vi "Without DRAM Packing Test Compile.vi"() -> ()   [LabVIEW 2013]
doc: "This is the FPGA VI for the 10-Tap 8-Bit Camera with DRAM example. This example demonstrates how to acquire images from a 10-tap, 8-bit, extended configuration, Camera Link camera and transfer the images to the host. This example supports area scan and line scan cameras for both continuous and finite acquisitions.\n\nThis example also demonstrates the use of DRAM as a frame buffer for very high speed acquisitions. Data packing and flow-control are also employed to maximize use of the available DRAM and FIFOs in terms of both memory space and performance.\n\nAdditionally, the example demonstrates the serial server, which allows third-party camera configuration utilities to communicate with the camera using the Camera Link serial interface while this VI is running."
uses:
  <vilib>/rvi/DataTransferAndStorage/Container/XNode/niFpgaContainer.xnode
  <vilib>/Platform/TimedLoop/XDataNode/XDataNode.xnode
  <vilib>/Platform/TimedLoop/XDataNode/timing_clust.ctl
  <vilib>/Platform/TimedLoop/XDataNode/XDNodeRunTimeDep.lvlib
  <vilib>/Platform/TimedLoop/XDataNode/wakeup.ctl
  <vilib>/Platform/TimedLoop/XDataNode/nitl_modes.ctl
  <vilib>/eio/EIONode/EIONode.xnode
  <vilib>/rvi/eio/common/nirviEmuTemplateMethod_errors.vi
  <vilib>/rvi/FIFO/Fifo_Resource/nirvififoEmulationGetNumberOfElementsToRead.vi
  <vilib>/rvi/interface/RandomDataEmulation/nirviRandomDataFpgaReadWriteTemplate.vi
  <vilib>/rvi/FIFO/Fifo_Resource/nirvififoEmulationRead.vi
  <vilib>/rvi/FIFO/Fifo_Resource/nirvififoEmulationWrite.vi
  Common/CL Data to Pixels/10 Tap 8-Bit.vi
  FPGA/10-Tap Data/10-Tap Conversion Enum.ctl
  FPGA/Globals/Accumulated Sector Intensity.vi
  FPGA/Globals/Pixel Location Global.vi
  FPGA/Globals/Wing Square Wave Frequency Global.vi
  FPGA/Globals/Sector Parameter Global.vi
  Common/CL Signal Mapping.ctl
  Common/CL Configuration.ctl
  FPGA/Sector/Accumulate/Sector Parameter Cluster.ctl
panel:
  in  "[Average BG Intensity]":u8[](array[numeric])=[0, 0, 0, 0, 0, 0, 0, 0, 0, 0, 0, 0, 0, 0, 0, 0, 0, 0, 0, 0, 0, 0, 0, 0, 0, 0, 0, 0, 0, 0, 0, 0]
  in  "Sector Threshold":u8
  in  "# of Frames to Average":u8
  in  "Sector Parameters Right":T1={"Start Angle"=0.13543701171875, "End Angle"=0.30462646484375, "Inner Radius"=309, "Outter Radius"=405, "Hinge X"=1106, "Hinge Y"=803, "NumWingSectors"=8}
  in  "Sector Parameters Left":T1={"Start Angle"=0.6541748046875, "End Angle"=0.856201171875, "Inner Radius"=309, "Outter Radius"=405, "Hinge X"=947, "Hinge Y"=829, "NumWingSectors"=8}
  in  "Sim":bool=TRUE
  in  "CL Config.Configuration":T2=enum."Full"
  in  "CL Config.Signal Mapping":T3=enum."Basler 10-tap"
  in  "CL Config.Line Scan":bool
  in  "CL Config.DVAL Active High":bool=TRUE
  in  "CL Config.LVAL Active High":bool=TRUE
  in  "CL Config.FVAL Active High":bool=TRUE
  in  "CL Config.Spare Active High":bool=TRUE
  in  "Acq Control.Line Scan Height":u32
  in  "Acq Control.Frames To Acq":u32
  in  "Acq Control.Acquire":bool
  in  "Acq Control.Cancel Acq":bool
  in  "Acq Control.Ignore DVAL":bool
  in  "Acq Control.Initialize":bool
  out "Acq Status.Acq In Progress":bool
  out "Acq Status.Clocks Per Line":u32
  out "Acq Status.Frames Acq'd":u32
  out "Acq Status.Lines Per Frame":u32
  out "Acq Status.DMA Write Timeout":bool
  out "Acq Status.Initialized":bool
  in  "UART.Baud Rate":u8
  in  "UART.Transmit":bool
  in  "UART.Tx Data":u8[](array[numeric])=[0, 0, 0, 0, 0, 0, 0, 0, 0, 0] format="%02x"
  in  "UART.Set Baud Rate":bool
  in  "UART.Byte Mode":bool=TRUE
  out "UART.Rx Ready":bool
  out "UART.Break Indicator":bool
  out "UART.Framing Error":bool
  out "UART.Overrun Error":bool
  out "UART.Tx Ready":bool
  out "UART.Rx Data":u8 format="%02x"
  in  "UART.Receive":bool
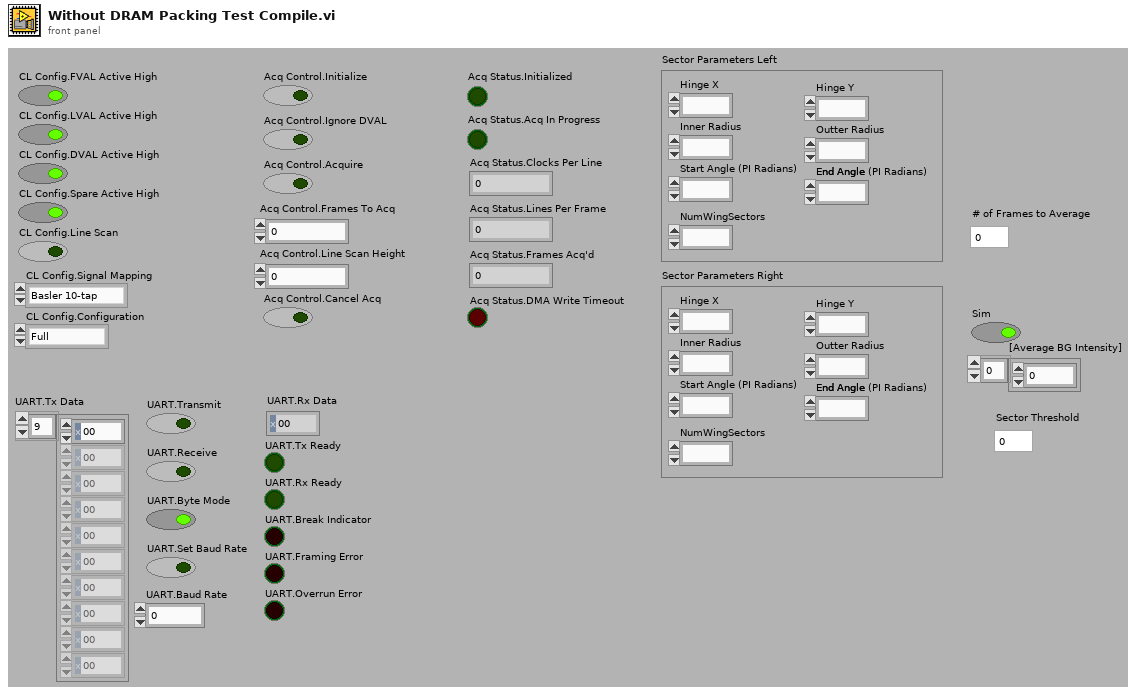
[diagram p1: front panel]
types:
  T1 = typedef "Sector Parameter Cluster.ctl" = cluster{"Start Angle":fxp<+/-,17,2>, "End Angle":fxp<+,17,3>, "Inner Radius":u16, "Outter Radius":u16, "Hinge X":u16, "Hinge Y":u16, "NumWingSectors":u8}
  T2 = typedef "CL Configuration.ctl" = enum8{"Base", "Medium", "Full"}
  T3 = typedef "CL Signal Mapping.ctl" = enum8{"Standard", "Basler 10-tap", "Vosskühler 10-tap"}
  T4 = typedef "XDNodeRunTimeDep.lvlib/timing_clust.ctl" = cluster{"Expected End [f-1]":u64, "Actual End [f-1]":u64, "Finished Late? [f-1]":bool, "Expected End [i-1]":u64, "Actual End [i-1]":u64, "Finished Late? [i-1]":bool, "Expected Start [i]":u64, "Actual Start [i]":u64, "Expected Start [f]":u64, "Actual Start [f]":u64, "Source Name":string, "Structure Name":string, "Period":i64, "Deadline":i64, "Offset":i64, "Start":i64, "Priority":i32, "Timeout":i32, "Mode":T5, "Wakeup Reason":T6, "Error":errorcluster, "Source Type":string, "Secondary Source Type":string, "Global End Time":u64, "Global Start Time":u64, "Frame Duration":u64, "Iteration Duration":u64, "Assigned CPU":i32, "I/O Scan Engine Mode":u32}
  T5 = typedef "XDNodeRunTimeDep.lvlib/nitl_modes.ctl" = enum32{"No Change", "Process missed periods, maintain original phase", "Discard missed periods, maintain original phase", "Process missed periods, ignore original phase", "Discard missed periods, ignore original phase"}
  T6 = typedef "XDNodeRunTimeDep.lvlib/wakeup.ctl" = enum32{"Normal", "Aborted", "Asynchronous wakeup", "Timing source error", "Timed loop error", "Timeout"}
  T7 = typedef "10-Tap Conversion Enum.ctl" = enum16{"10-Tap to 16 and 64", "16 and 64 to 10-Tap"}
  T8 = cluster{"Enables Valid":bool, "Frame Valid":bool, "Line Valid":bool, "Data Valid":bool}
  T9 = typedef "10-Tap 8-bit Cluster.ctl" = cluster{"Pixel 0":u8, "Pixel 1":u8, "Pixel 2":u8, "Pixel 3":u8, "Pixel 4":u8, "Pixel 5":u8, "Pixel 6":u8, "Pixel 7":u8, "Pixel 8":u8, "Pixel 9":u8}
  T10 = cluster{"Tx Data":u8[], "Transmit":bool, "Receive":bool, "Byte Mode":bool, "Set Baud Rate":bool, "Baud Rate":u8}
  T11 = cluster{"Rx Data":u8, "Turn Off Transmit":bool, "Turn Off Receive":bool, "Turn Off Set Baud Rate":bool, "Tx Ready":bool, "Rx Ready":bool, "Break Indicator":bool, "Framing Error":bool, "Overrun Error":bool}
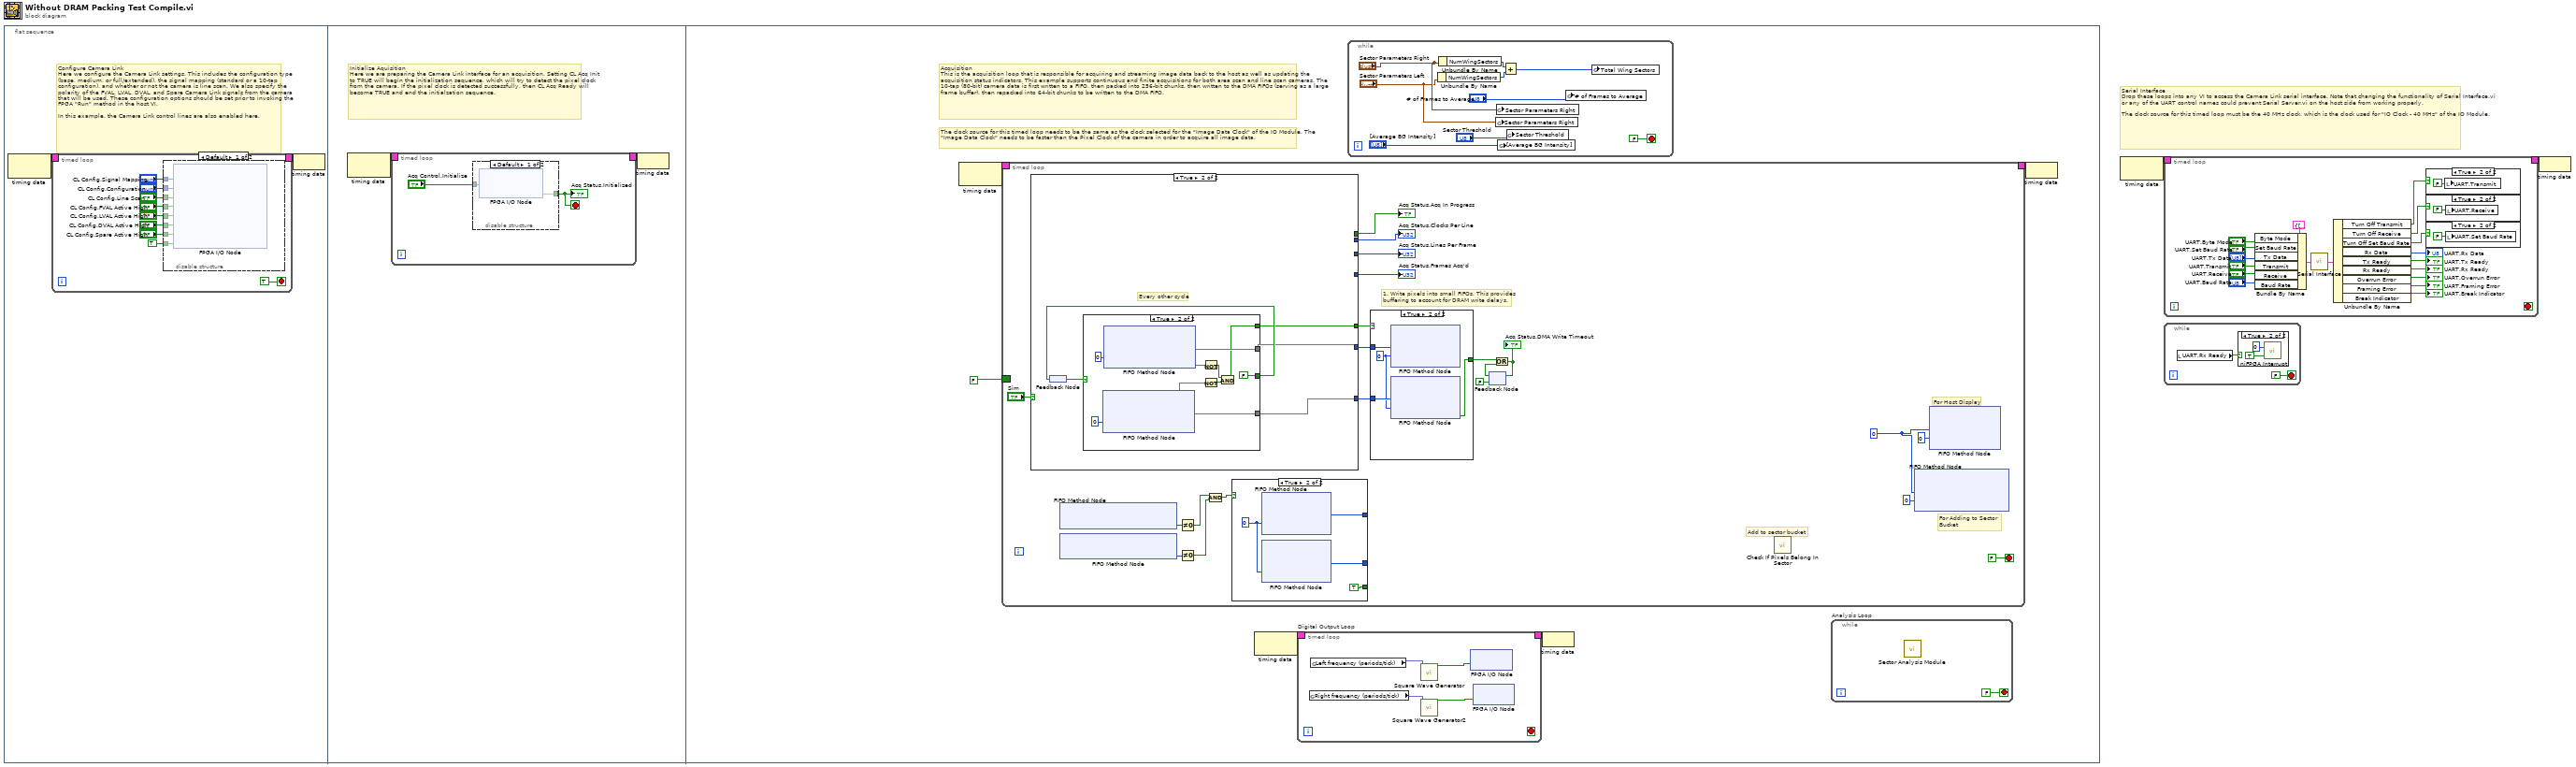
[diagram p0: block diagram]
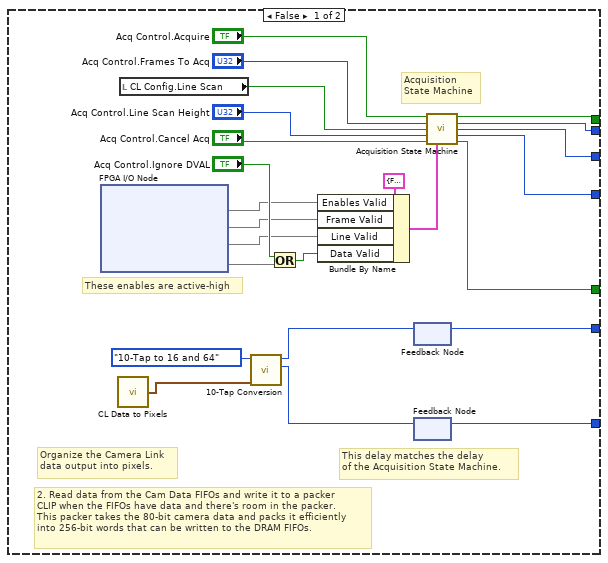
[diagram p8: hidden frame]
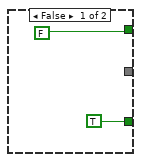
[diagram p9: hidden frame]
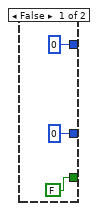
[diagram p10: hidden frame]
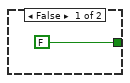
[diagram p11: hidden frame]
diagram:
  # "Serial Interface\nDrop these loops into any VI to access the Camera Link serial interface. Note that changing the functionality of Serial Interface.vi or any of the UART control names could prevent Serial Server.vi on the host side from working properly.\n\nThe clock source for this timed loop must be the 40 MHz clock, which is the clock used for \"IO Clock - 40 MHz\" of the IO Module."
  n1 = flat-sequence {
    frame #0 {
      # "Configure Camera Link\nHere we configure the Camera Link settings. This includes the configuration type (base, medium, or full/extended), the signal mapping (standard or a 10-tap configuration), and whether or not the camera is line scan. We also specify the polarity of the FVAL, LVAL, DVAL, and Spare Camera Link signals from the camera that will be used. These configuration options should be set prior to invoking the FPGA \"Run\" method in the host VI.\n\nIn this example, the Camera Link control lines are also enabled here."
      n2 = node-c288() -> (w4:T4)  [unwired: 1 in]
      n3 = timed-loop {
        timing: w4 -> [_]
        timing-out: [_] -> w3
        stop <- TRUE stop-if-true
        n4 = disable-structure shown="Default" {
          disable-tunnel: "CL Config.FVAL Active High" -> [w21 _]
          disable-tunnel: "CL Config.LVAL Active High" -> [w20 _]
          disable-tunnel: "CL Config.DVAL Active High" -> [w19 _]
          disable-tunnel: "CL Config.Spare Active High" -> [w18 _]
          disable-tunnel: "CL Config.Signal Mapping" -> [w17 _]
          disable-tunnel: "CL Config.Configuration" -> [w16 _]
          disable-tunnel: "CL Config.Line Scan" -> [w15 _]
          disable-tunnel: TRUE ("IO Module\\CL Control Enable") -> [w14 _]
          frame condition #0 {
            n5 = xnode "FPGA I/O Node"("CL Set Signal Mapping"=w17, "CL Set Configuration"=w16, "CL Set Line Scan"=w15, "CL Set FVAL Active High"=w21, "CL Set LVAL Active High"=w20, "CL Set DVAL Active High"=w19, "CL Set Spare Active High"=w18, "CL Control Enable"=w14) -> ()  [unwired: 8 in, 8 out]
          }
          frame condition #1 (active) {
          }
        }
      }
      n6 = node-c288(w3) -> ()
    }
    frame #1 {
      # "Initialize Aquisition\nHere we are preparing the Camera Link interface for an acquisition. Setting CL Acq Init to TRUE will begin the initialization sequence, which will try to detect the pixel clock from the camera. If the pixel clock is detected successfully, then CL Acq Ready will become TRUE and end the initialzation sequence."
      n7 = node-c288() -> (w27:T4)  [unwired: 1 out]
      n8 = timed-loop {
        timing: w27 -> [_]
        timing-out: [_] -> w26
        stop <- w28 stop-if-true
        n9 = disable-structure shown="Default" {
          disable-tunnel: "Acq Control.Initialize" -> [w31 w32]
          disable-tunnel: [w30 w32] -> w28
          frame condition #0 {
            n10 = xnode "FPGA I/O Node"("CL Acq Init"=w31) -> ("CL Acq Ready"=w30)  [unwired: 2 in, 2 out]
          }
          frame condition #1 (active) {
          }
        }
        "Acq Status.Initialized" <- w28
      }
      n11 = node-c288(w26) -> ()
    }
    frame #2 {
      # "The clock source for this timed loop needs to be the same as the clock selected for the \"Image Data Clock\" of the IO Module. The \"Image Data Clock\" needs to be faster than the Pixel Clock of the camera in order to acquire all image data."
      # "Acquisition\nThis is the acquisition loop that is responsible for acquiring and streaming image data back to the host as well as updating the acquisition status indicators. This example supports continuous and finite acquisitions for both area scan and line scan cameras. The 10-tap (80-bit) camera data is first written to a FIFO, then packed into 256-bit chunks, then written to the DMA FIFOs (serving as a large frame buffer), then repacked into 64-bit chunks to be written to the DMA FIFO."
      n12 = node-c288() -> (w41:T4)  [unwired: 1 in]
      n13 = timed-loop {
        timing: w41 -> [_]
        timing-out: [_] -> w40
        border: FALSE -> [_]
        stop <- FALSE stop-if-true
        w60 = u64 0 ("Element")
        # "For Adding to Sector \nBucket"
        # "For Host Display"
        # "Add to sector bucket"
        # "1. Write pixels into small FIFOs. This provides\nbuffering to account for DRAM write delays."
        n14 = case shown="True" "Sim" {
          tunnel: [w104 w105] -> w80
          tunnel: [w103 w106] -> w75
          tunnel: [w85 w108] -> w67
          tunnel: [w89 _] -> w66
          tunnel: [w88 _] -> w65
          tunnel: [w87 _] -> w64
          tunnel: [w86 _] -> w63
          frame False {
            # "These enables are active-high"
            # "Acquisition\nState Machine"
            # "2. Read data from the Cam Data FIFOs and write it to a packer\nCLIP when the FIFOs have data and there's room in the packer.\nThis packer takes the 80-bit camera data and packs it efficiently\ninto 256-bit words that can be written to the DRAM FIFOs."
            # "Organize the Camera Link\ndata output into pixels."
            # "This delay matches the delay\nof the Acquisition State Machine."
            n15 = xnode "FPGA I/O Node"() -> ("CL Output Valid"=w93, "CL Frame Valid"=w94, "CL Line Valid"=w95, "CL Data Valid"=w98)  [unwired: 4 in, 4 out]
            n16 = call-poly "CL Data to Pixels.vi"() -> ("Pixels"=w81:T9)  [unwired: 1 in]
            n17 = local read "CL Config.Line Scan"() -> (w101:bool)
            n18 = call "10-Tap Conversion.vi"("10 Tap In"=w81, "Operation"=10-Tap_Conversion_Enum."10-Tap to 16 and 64") -> ("64 Bit Out"=w82:u64, "16 Bit Out"=w83:u16)  [unwired: 7 in, 1 out]
            n19 = Or(x="Acq Control.Ignore DVAL", y=w98) -> (x .or. y?=w99:bool)
            n20 = Bundle By Name(cluster=T8 {"Enables Valid"=FALSE, "Frame Valid"=FALSE, "Line Valid"=FALSE, "Data Valid"=FALSE} ("Enables"), "Enables Valid"=w93, "Frame Valid"=w94, "Line Valid"=w95, "Data Valid"=w99) -> (w96:T8)
            n21 = feedback #1() -> (w103:u16)  [unwired: 1 in]
            n22 = feedback-in #1(w83) -> ()
            n23 = feedback #2() -> (w104:u64)  [unwired: 1 in]
            n24 = feedback-in #2(w82) -> ()
            n25 = call "Acquisition State Machine.vi"("Acquire"="Acq Control.Acquire", "Frames to Acquire"="Acq Control.Frames To Acq", "Line Scan"=w101, "Line Scan Height"="Acq Control.Line Scan Height", "Cancel Acq"="Acq Control.Cancel Acq", "Enables"=w96) -> ("Acq In Progress"=w89:bool, "Num Clocks Per Line"=w88:u32, "Num Lines Per Frame"=w87:u32, "Num Frames Acq'd"=w86:u32, "Capture Cycle"=w85:bool)  [unwired: 4 in, 1 out]
          }
          frame True {
            # "Every other cycle"
            n26 = feedback #3() -> (w107:bool)
            n27 = case shown="True" w107 {
              tunnel: [_ w121] -> w106
              tunnel: [_ w120] -> w105
              tunnel: [FALSE w113] -> w108
              tunnel: [TRUE FALSE] -> w109
              frame False {
              }
              frame True {
                n28 = xnode ("FIFO Method Node")("Timeout"=0) -> ("Element"=w120, "Timed Out?"=w116)  [unwired: 1 in, 1 out]
                n29 = xnode ("FIFO Method Node")("Timeout"=0) -> ("Element"=w121, "Timed Out?"=w117)  [unwired: 1 in, 1 out]
                n30 = Not(x=w117) -> (.not. x?=w115:bool)
                n31 = Not(x=w116) -> (.not. x?=w114:bool)
                n32 = And(x=w115, y=w114) -> (x .and. y?=w113:bool)
              }
            }
            n33 = feedback-in #3(w109) -> ()
          }
        }
        "Acq Status.Frames Acq'd" <- w63
        "Acq Status.Lines Per Frame" <- w64
        "Acq Status.Clocks Per Line" <- w65
        "Acq Status.Acq In Progress" <- w66
        n34 = xnode ("FIFO Method Node")() -> ("Number of Elements to Read"=w74:u32)  [unwired: 1 in, 1 out]
        n35 = xnode ("FIFO Method Node")() -> ("Number of Elements to Read"=w73:u32)  [unwired: 1 in, 1 out]
        n36 = Not Equal To 0?(x=w74) -> (x != 0?=w71:bool)
        n37 = Not Equal To 0?(x=w73) -> (x != 0?=w70:bool)
        n38 = Compound Arithmetic op=AND(w71, w70) -> (w72:bool)
        n39 = case shown="True" w72 {
          tunnel: [u16 0 ("Element") w128] -> _
          tunnel: [u64 0 ("Element") w127] -> _
          tunnel: [FALSE TRUE] -> _
          frame False {
          }
          frame True {
            w126 = 0 ("Timeout")
            n40 = xnode ("FIFO Method Node")("Timeout"=w126) -> ("Element"=w128:u16)  [unwired: 1 in, 2 out]
            n41 = xnode ("FIFO Method Node")("Timeout"=w126) -> ("Element"=w127:u64)  [unwired: 1 in, 2 out]
          }
        }
        n42 = case shown="True" w67 {
          tunnel: [FALSE ("Timed Out?") w132] -> w78
          tunnel: w80 -> [_ w133]
          tunnel: w75 -> [_ w131]
          frame False {
          }
          frame True {
            w130 = 0 ("Timeout")
            n43 = xnode ("FIFO Method Node")("Element"=w131, "Timeout"=w130) -> ()  [unwired: 1 in, 2 out]
            n44 = xnode ("FIFO Method Node")("Element"=w133, "Timeout"=w130) -> ("Timed Out?"=w132:bool)  [unwired: 1 in, 1 out]
          }
        }
        n45 = feedback #4(FALSE) -> (w77:bool)
        n46 = Or(x=w78, y=w77) -> (x .or. y?=w76:bool)
        "Acq Status.DMA Write Timeout" <- w76
        n47 = feedback-in #4(w76) -> ()
        n48 = call "Check If Pixels Belong In Sector.vi"() -> ()  [unwired: 11 in, 1 out]
        n49 = xnode ("FIFO Method Node")("Element"=w60, "Timeout"=0) -> ()  [unwired: 1 in, 2 out]
        n50 = xnode ("FIFO Method Node")("Element"=w60, "Timeout"=0) -> ()  [unwired: 1 in, 2 out]
      }
      n51 = node-c288() -> (w38:T4)  [unwired: 1 in]
      n52 = timed-loop "Digital Output Loop" {
        timing: w38 -> [_]
        timing-out: [_] -> w37
        stop <- _ stop-if-true
        n53 = global read "Wing Square Wave Frequency Global.vi" "Right frequency (periods/tick)"() -> (w52:fxp<+,32,0>)
        n54 = global read "Wing Square Wave Frequency Global.vi" "Left frequency (periods/tick)"() -> (w53:fxp<+,32,0>)
        n55 = call "Square Wave Generator"("frequency (periods/tick)"=w53) -> ("square wave out"=w55:bool)  [unwired: 14 in]
        n56 = call "Square Wave Generator2"("frequency (periods/tick)"=w52) -> ("square wave out"=w54:bool)  [unwired: 14 in]
        n57 = xnode "FPGA I/O Node"("TTL 0"=w55) -> ()  [unwired: 1 in, 1 out]
        n58 = xnode "FPGA I/O Node"("TTL 1"=w54) -> ()  [unwired: 1 in, 1 out]
      }
      n59 = while {
        stop <- FALSE stop-if-true
        n60 = Unbundle By Name("Sector Parameters Left") -> ("NumWingSectors"=w48:u8)
        n61 = Unbundle By Name("Sector Parameters Right") -> ("NumWingSectors"=w49:u8)
        n62 = global write "Sector Parameter Global.vi" "Sector Parameters Right"("Sector Parameters Left") -> ()
        n63 = global write "Sector Parameter Global.vi" "Sector Parameters Right"("Sector Parameters Right") -> ()
        n64 = global write "Sector Parameter Global.vi" "[Average BG Intensity]"("[Average BG Intensity]") -> ()
        n65 = Add(x=w49, y=w48) -> (x+y=w47:u8)
        n66 = global write "Sector Parameter Global.vi" "Sector Threshold"("Sector Threshold") -> ()
        n67 = global write "Pixel Location Global.vi" "# of Frames to Average"("# of Frames to Average") -> ()
        n68 = global write "Accumulated Sector Intensity.vi" "Total Wing Sectors"(w47) -> ()
      }
      n69 = node-c288(w37) -> ()
      n70 = while "Analysis Loop" {
        stop <- FALSE stop-if-true
        n71 = call "Sector Analysis Module.vi"() -> ()  [unwired: 7 in, 5 out]
      }
      n72 = node-c288(w40) -> ()
    }
  }
  n73 = node-c288() -> (w2:T4)  [unwired: 1 out]
  n74 = timed-loop {
    timing: w2 -> [_]
    timing-out: [_] -> w1
    stop <- _ stop-if-true
    n75 = Bundle By Name(cluster=T10 {"Tx Data"=[0, 0, 0, 0, 0, 0, 0, 0, 0, 0], "Transmit"=FALSE, "Receive"=FALSE, "Byte Mode"=TRUE, "Set Baud Rate"=FALSE, "Baud Rate"=0} ("UART Inputs"), "Byte Mode"="UART.Byte Mode", "Set Baud Rate"="UART.Set Baud Rate", "Tx Data"="UART.Tx Data", "Transmit"="UART.Transmit", "Receive"="UART.Receive", "Baud Rate"="UART.Baud Rate") -> (w138:T10)
    n76 = call "Serial Interface.vi"("UART Inputs"=w138) -> ("UART Outputs"=w150:T11)
    n77 = Unbundle By Name(w150) -> ("Turn Off Transmit"=w143:bool, "Turn Off Receive"=w144:bool, "Turn Off Set Baud Rate"=w140:bool, "Rx Data"=→"UART.Rx Data":u8, "Tx Ready"=→"UART.Tx Ready":bool, "Rx Ready"=→"UART.Rx Ready":bool, "Overrun Error"=→"UART.Overrun Error":bool, "Framing Error"=→"UART.Framing Error":bool, "Break Indicator"=→"UART.Break Indicator":bool)
    n78 = case shown="True" w143 {
      frame False {
      }
      frame True {
        n79 = local write "UART.Transmit"(FALSE ("UART.Transmit")) -> ()
      }
    }
    n80 = case shown="True" w144 {
      frame False {
      }
      frame True {
        n81 = local write "UART.Receive"(FALSE ("UART.Receive")) -> ()
      }
    }
    n82 = case shown="True" w140 {
      frame False {
      }
      frame True {
        n83 = local write "UART.Set Baud Rate"(FALSE ("UART.Receive")) -> ()
      }
    }
  }
  n84 = while {
    stop <- FALSE stop-if-true
    n85 = local read "UART.Rx Ready"() -> (w162:bool)
    n86 = case shown="True" w162 {
      frame False {
      }
      frame True {
        n87 = call <vilib>:"niFPGA Interrupt.vi"("Wait Until Cleared (F)"=TRUE ("Wait Until Cleared"), "IRQ Number (0)"=u8 0 ("IRQ Number")) -> ()  [unwired: 1 in]
      }
    }
  }
  n88 = node-c288(w1) -> ()
